vi "xeva-startAcquisition.vi"(3 "error in (no error)":errorcluster, 5 "xeva-camref":T1) -> (0 "error out":errorcluster, 1 "xeva-acquiring":bool, 2 "xeva-camref":T1)   [LabVIEW 2015]
doc: "This example shows how to open the camera, grab frames and display them on the control-panel. To get a better visualisation the histogram is spread."
uses:
  <vilib>/Xenics Infrared Solutions/Xeneth LabVIEW API/VIs/Controls/Camara.ctl
  <vilib>/Xenics Infrared Solutions/Xeneth LabVIEW API/Xeneth.lvlib
panel:
  out "error cluster":bool[](array[boolean])
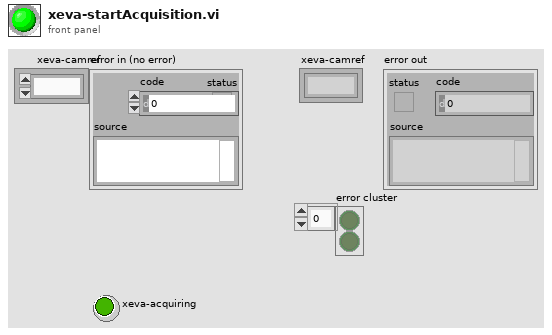
[diagram p1: front panel]
types:
  T1 = typedef "Xeneth.lvlib/Camara.ctl" = refnum<k1>
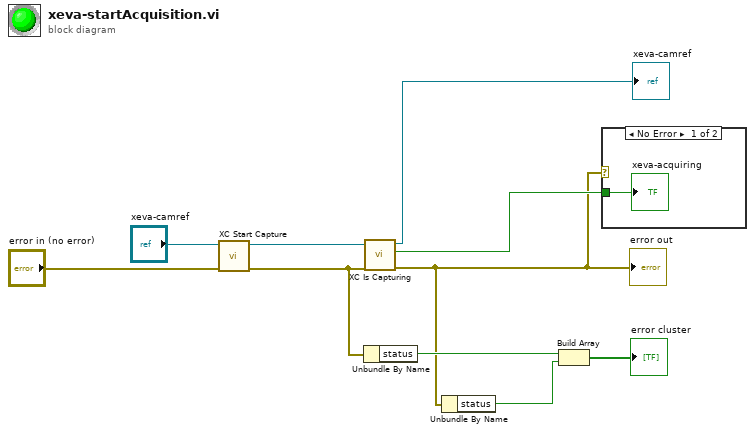
[diagram p0: block diagram]
diagram:
  n1 = call <vilib>:"XC Start Capture.vi"("error in (no error)"="error in (no error)", "Cam Ref"="xeva-camref") -> ("error out"=w8:errorcluster, "Cam Ref Out"=w4:T1)  [unwired: 8 in]
  n2 = Unbundle By Name(w8) -> ("status"=w7:bool)
  n3 = call <vilib>:"XC Is Capturing.vi"("error in (no error)"=w8, "Cam Ref"=w4) -> ("error out"=w1:errorcluster, "IsCapturing"=w2:bool, "Cam Ref Out"=→"xeva-camref":T1)  [unwired: 7 in]
  "error out" <- w1
  n4 = Unbundle By Name(w1) -> ("status"=w6:bool)
  n5 = Build Array(w7, w6) -> (→"error cluster":bool[])
  n6 = case shown="No Error" w1 {
    tunnel: w2 -> [w11 _]
    frame No Error {
      "xeva-acquiring" <- w11
    }
    frame Error {
    }
  }
